vi "消息通知.vi"() -> ()   [LabVIEW 2018]
panel:
  in  "400nm对应步数":dbl
  out "disableUI":bool
  out "moveComplete":bool
  out "moveStopped":bool
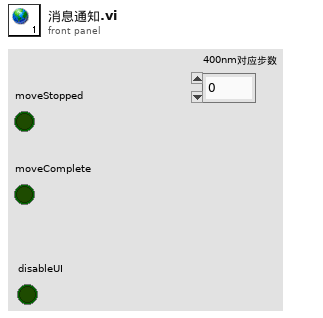
[diagram p1: front panel]
diagram:
